vi "Navigation_Main_r1.4 (less sub vis).vi"() -> ()   [LabVIEW 2015]
uses:
  <vilib>/myRIO/Common/Instrument Driver Framework/Utilities/typedefs/Generic FPGA Reference.ctl
  <vilib>/myRIO/Common/Instrument Driver Framework/Utilities/typedefs/myRIO v1.0 Reference.ctl
  <vilib>/myRIO/Common/Instrument Driver Framework/Utilities/typedefs/Hardware Version Enum.ctl
  <vilib>/myRIO/Common/Instrument Driver Framework/Utilities/typedefs/myRIO Generic Hardware Reference.ctl
  <vilib>/userdefined/High Color/nirio_resource_hc.ctl
  <vilib>/myRIO/Instrument Drivers/Onboard IO/PWM/typedefs/PWM Configuration.ctl
  <vilib>/myRIO/Instrument Drivers/Onboard IO/PWM/PWM.lvlib
  <vilib>/myRIO/Common/Instrument Driver Framework/myRIO v1.0/PWM/typedefs/PWM Channels Enum.ctl
  <vilib>/myRIO/Instrument Drivers/Onboard IO/PWM/typedefs/PWM Reference.ctl
  <vilib>/myRIO/Instrument Drivers/Onboard IO/PWM/vis/myRIO PWM Open.xnode
  <vilib>/myRIO/Common/Instrument Driver Framework/myRIO v1.0/PWM/vis/myRIO v1.1 Open PWM.vi
  <vilib>/rvi/interface/nirviOpenFPGA/nirviOpenFPGA.xnode
  <vilib>/myRIO/Instrument Drivers/Utilities/Utilities.lvlib
  <vilib>/rvi/interface/nirviReadWriteControl/nirviReadWriteControl.xnode
  NiFpgaLv.dll
  <vilib>/Utility/error.llb/Error Cluster From Error Code.vi
  <vilib>/rvi/interface/Simulation/niFpgaSimulationCallBeginRW.vi
  <vilib>/rvi/errors/niLvFpgaAdjustHostInterfaceError.vi
  Navi/E/FPGA Bitfiles/NavigationProjec_FPGATarget2_FPGAMainNavigati_PWPHW8gwDxI.lvbitx
  <vilib>/FPGAPlugInAG/myRIO-1900/niLvFpga_Open_myRIO-1900.vi
  <vilib>/rvi/interface/common/dynamic/niFpgaDynamicAddResources.vi
  <vilib>/addons/control/pid/NI_PID_pid.lvlib
  <vilib>/addons/control/pid/pid.llb/PID (DBL).vi
panel:
  out "Avg Right Step":dbl
  out "Avg Left Step":dbl
  out "distance step 2":dbl
  in  "Reset X Y 3":dbl=1.0
  out "Avg Left Dist. New":dbl
  out "Avg Right Dist. New":dbl
  in  "distance step":dbl
  out "step y":dbl
  out "step x":dbl
  out "y traveled new":dbl
  out "x traveled new":dbl
  out "Y traveled old":dbl format="%#_13g"
  out "X traveled old":dbl format="%#_13g"
  out "phi step":dbl
  in  "Reset X Y 2":dbl=1.0
  out "y position":dbl
  out "x position":dbl
  out "phi current":dbl
  out "Phi Current":dbl format="%#_13g"
  out "Desired Y Velocity u2":dbl format="%#_13g"
  out "Desired X Velocity u1":dbl format="%#_13g"
  out "Phi desired":dbl
  out "Omega":dbl format="%.2f"
  out "Desired Velocity":dbl
  in  "omega and angular velocity calc input array 2":dbl[](array[numeric])
  out "robot desired velocity x component\n u1 (ft/s)":dbl
  out "x goal":dbl
  out "x start":dbl
  out "robot desired velocity y component\n u2 (ft/s)":dbl
  out "Y Goal":dbl
  out "Y Position":dbl
  out "Tick Count(mSec) 2":u32 caption="Tick Count(mSec)"
  out "Left Setpoint":dbl
  out "Right Setpoint":dbl
  out "Reset X Y":dbl
  out "Scale":dbl=1.0
  out "x traveled":dbl
  out "v right wheel":dbl
  out "v left wheel":dbl
  out "max v":dbl
  in  "loc_x":dbl
  out "x delta":dbl
  out "x position camera":dbl
  out "encoder step sub vi output":dbl[](array[numeric])
  out "Avg R Dist New":dbl
  out "Avg R Step":dbl
  out "Avg L Dist New":dbl
  out "Avg L Step":dbl
  in  "Avg R Dist Old":dbl
  in  "Avg L Dist Old":dbl
  out "encoder sub vi input array":dbl[](array[numeric])
  out "x & y position output array":dbl[](array[numeric])
  out "x & y position input array":dbl[](array[numeric])
  in  "x traveled old":dbl
  in  "y traveled old":dbl
  in  "phi old":dbl
  in  "Phi Current":dbl format="%#_13g"
  out "Wheel  PID SetPoint input Array":dbl[](array[numeric])
  out "Wheel  PID SetPoint output Array":dbl[](array[numeric])
  in  "Goal Position Y":dbl=5.0
  out "track width(ft)":dbl=4.0
  out "RM Distance (ft)":dbl
  out "RR Distance (ft)":dbl
  out "LF Distance (ft)":dbl
  out "LM Distance (ft)":dbl
  out "RF Distance (ft)":dbl
  out "LR Distance (ft)":dbl
  in  "Start Position Y":dbl=5.0
  in  "Goal Position X":dbl=5.0
  in  "Start Position X":dbl=1.0
  in  "All Stop":bool
  in  "Left Side PID Gains":T1={"proportional gain (Kc)"=0.002, "integral time (Ti, min)"=7e-07, "derivative time (Td, min)"=0.0} {"derivative time (Td, min)" format="%.8f"; "integral time (Ti, min)" format="%.8f"; "proportional gain (Kc)" format="%.8f"}
  in  "Left Side Output Range":cluster{"output high":dbl, "output low":dbl}={"output high"=0.13333, "output low"=-0.13333} {"output low" format="%.5f"; "output high" format="%.5f"}
  in  "Right Side PID Gains":T1={"proportional gain (Kc)"=0.002, "integral time (Ti, min)"=7e-07, "derivative time (Td, min)"=0.0} {"derivative time (Td, min)" format="%.8f"; "integral time (Ti, min)" format="%.8f"; "proportional gain (Kc)" format="%.8f"}
  in  "Right Side Output Range":cluster{"output high":dbl, "output low":dbl}={"output high"=0.13333, "output low"=-0.13333} {"output low" format="%.5f"; "output high" format="%.5f"}
  out "Left PWM":dbl
  out "Right PWM":dbl
  out "LF Rot Velocity (rot/s)":dbl
  out "LM Rot Velocity (rot/s)":dbl
  out "LR Rot Velocity (rot/s)":dbl
  out "RR Rot Velocity (rot/s)":dbl
  out "RM Linear Velocity (rot/s)":dbl
  out "RF Linear Velocity (rot/s)":dbl
  in  "Encoder Reset":bool
  out "SYS.SELECTA":u8 format="%08b"
  out "ENC.B_c.CNTR":i32
  out "ENC.B_b.CNTR":i32
  out "ENC.B_a.CNTR":i32
  out "ENC.A_c.CNTR":i32
  out "ENC.A_b.CNTR":i32
  out "ENC.A_a.CNTR":i32
  out "Current Rot Velocity (rot/s)":T2(graph)
  # "Motor Control Parameters"
  # "Press Go when Start and Goal Are Set"
types:
  T1 = cluster{"proportional gain (Kc)":dbl, "integral time (Ti, min)":dbl, "derivative time (Td, min)":dbl}
  T2 = cluster{"Rotational Velocity (RPS)":dbl, "Rotational Velocity (RPS)":dbl, "Rotational Velocity (RPS)":dbl, "Rotational Velocity (RPS)":dbl, "Rotational Velocity (RPS)":dbl, "Rotational Velocity (RPS)":dbl}
  T3 = typedef "nirio_resource_hc.ctl" = tag
  T4 = typedef "Hardware Version Enum.ctl" = enum16{"Unknown", "myRIO-1900", "myRIO-1950", "roboRIO"}
  T5 = typedef "PWM.lvlib/PWM Reference.ctl" = cluster{"myRIO Reference":T6, "PWM Channels Enum":T9, "PWM Configuration":T10}
  T6 = typedef "myRIO Generic Hardware Reference.ctl" = cluster{"myRIO Model":T4, "myRIO Hardware Reference":T7}
  T7 = typedef "myRIO v1.0 Reference.ctl" = cluster{"Generic FPGA Reference":T8, "Allow multiple opens":bool}
  T8 = typedef "Generic FPGA Reference.ctl" = refnum<k20>
  T9 = typedef "PWM Channels Enum.ctl" = enum16{"Not Connected", "C/PWM0", "C/PWM1", "A/PWM0", "A/PWM1", "A/PWM2", "B/PWM0", "B/PWM1", "B/PWM2", "PWM/PWM0", "PWM/PWM1", "PWM/PWM2", "PWM/PWM3", "PWM/PWM4", "PWM/PWM5", "PWM/PWM6", "PWM/PWM7", "PWM/PWM8", "PWM/PWM9"}
  T10 = typedef "PWM.lvlib/PWM Configuration.ctl" = cluster{"Frequency":dbl, "Duty Cycle":dbl}
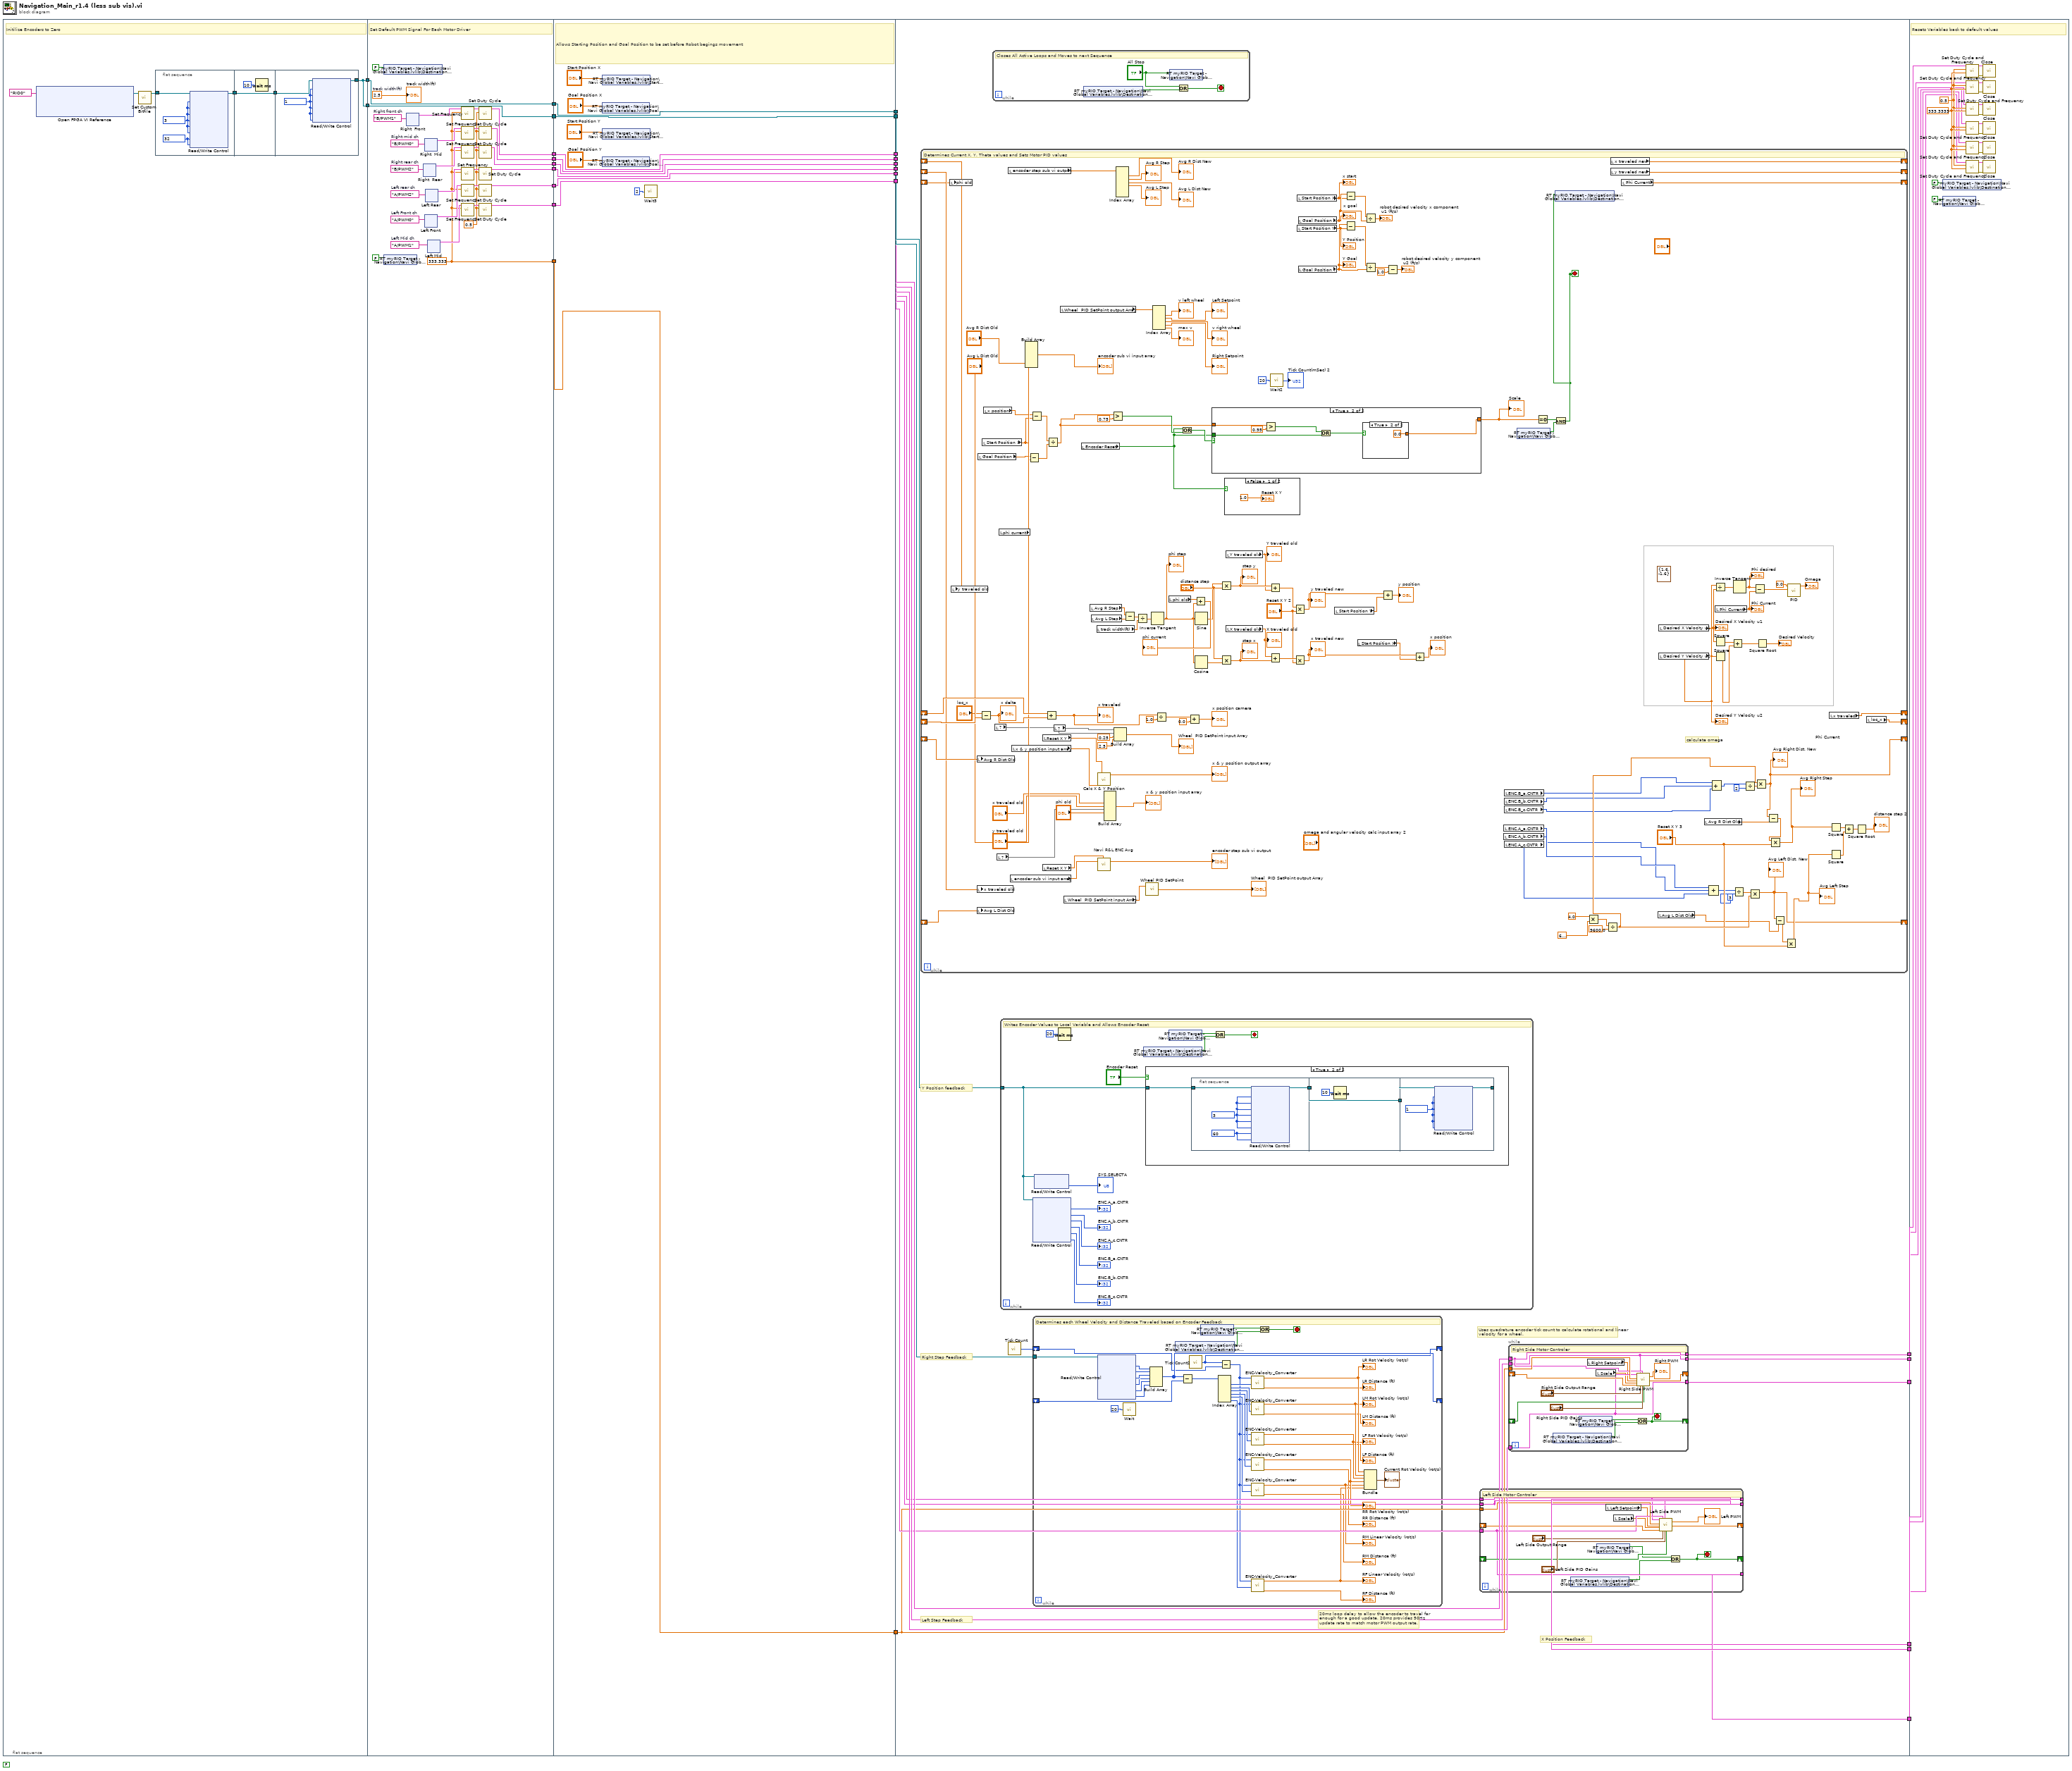
[diagram p0: block diagram]
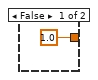
[diagram p2: hidden frame]
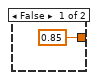
[diagram p3: hidden frame]
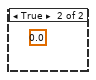
[diagram p4: hidden frame]
diagram:
  (unwired) FALSE ("stop")
  n1 = flat-sequence {
    tunnel: [w29] -> w26
    tunnel: [w29] -> w25
    tunnel: [w60] -> w24
    tunnel: [w55] -> w23
    tunnel: [w51] -> w22
    tunnel: [w50] -> w21
    tunnel: [w49] -> w20
    tunnel: [w48] -> w19
    tunnel: [w47] -> w18
    tunnel: [w46] -> w17
    tunnel: w26 -> [w45]
    tunnel: [w45] -> w16
    tunnel: w25 -> [w46]
    tunnel: w24 -> [w182]
    tunnel: [w182] -> w15
    tunnel: w23 -> [w181]
    tunnel: [w181] -> w14
    tunnel: w22 -> [w180]
    tunnel: [w180] -> w13
    tunnel: w21 -> [w169]
    tunnel: [w169] -> w12
    tunnel: w20 -> [w179]
    tunnel: [w179] -> w11
    tunnel: w19 -> [w178]
    tunnel: [w178] -> w10
    tunnel: w18 -> [w177]
    tunnel: [w177] -> w9
    tunnel: w17 -> [w176]
    tunnel: [w176] -> w8
    tunnel: w16 -> [w175]
    tunnel: [w175] -> w7
    tunnel: w15 -> [w189]
    tunnel: w14 -> [w190]
    tunnel: w13 -> [w195]
    tunnel: w12 -> [w194]
    tunnel: w11 -> [w193]
    tunnel: w10 -> [w192]
    tunnel: w9 -> [w191]
    tunnel: w8 -> [w197]
    tunnel: w7 -> [w196]
    tunnel: [w188] -> w6
    tunnel: [w187] -> w5
    tunnel: [w186] -> w4
    tunnel: [w185] -> w3
    tunnel: [w184] -> w2
    tunnel: [w183] -> w1
    tunnel: w6 -> [w461]
    tunnel: w5 -> [w460]
    tunnel: w4 -> [w459]
    tunnel: w3 -> [w458]
    tunnel: w2 -> [w457]
    tunnel: w1 -> [w456]
    frame #0 {
      # "Initilize Encoders to Zero"
      n2 = xnode "Open FPGA VI Reference"("resource name"=tag "RIO0") -> ("FPGA VI Reference Out"=w28:refnum<k20>)  [unwired: 1 in, 1 out]
      n3 = call <vilib>:"Set Custom Bitfile.vi"("Custom FPGA Reference In"=w28) -> ("Custom FPGA Reference Out"=w30:refnum<k20>)  [unwired: 9 in, 1 out]
      n4 = flat-sequence {
        tunnel: w30 -> [w35]
        tunnel: [w33] -> w32
        tunnel: w32 -> [w37]
        tunnel: [w37] -> w31
        tunnel: w31 -> [w40]
        tunnel: [w39] -> w29
        frame #0 {
          w34 = u8 32 ("SYS.SELECTA")
          w36 = u8 3 ("ENC.B_c.CNFG")
          n5 = xnode "Read/Write Control"("FPGA VI Reference In"=w35, "ENC.A_a.CNFG"=w36, "ENC.A_b.CNFG"=w36, "ENC.A_c.CNFG"=w36, "ENC.B_a.CNFG"=w36, "ENC.B_b.CNFG"=w36, "ENC.B_c.CNFG"=w36, "SYS.SELECTA"=w34, "SYS.SELECTB"=w34) -> ("FPGA VI Reference Out"=w33:refnum<k20>)  [unwired: 1 in, 1 out]
        }
        frame #1 {
          n6 = Wait (ms)(milliseconds to wait=u32 10) -> ()  [unwired: 1 out]
        }
        frame #2 {
          w41 = u8 1 ("ENC.B_c.CNFG")
          n7 = xnode "Read/Write Control"("FPGA VI Reference In"=w40, "ENC.A_a.CNFG"=w41, "ENC.A_b.CNFG"=w41, "ENC.A_c.CNFG"=w41, "ENC.B_a.CNFG"=w41, "ENC.B_b.CNFG"=w41, "ENC.B_c.CNFG"=w41) -> ("FPGA VI Reference Out"=w39:refnum<k20>)  [unwired: 1 in, 1 out]
        }
      }
    }
    frame #1 {
      w42 = 2.5  # track width(ft)
      w52 = 0.5 ("Duty Cycle")
      w60 = 333.333 ("Frequency [Hz]")
      w67 = tag "B/PWM2"  # Right rear ch
      w68 = tag "B/PWM0"  # Right mid ch
      w69 = tag "B/PWM1"  # Right front ch
      w70 = tag "A/PWM2"  # Left rear ch
      w71 = tag "A/PWM0"  # Left Front ch
      w72 = tag "A/PWM1"  # Left Mid ch
      # "Set Default PWM Signal For Each Motor Driver"
      n8 = shared-variable "RT myRIO Target - Navigation\\Navi Global Variables.lvlib\\Destination Reached"(FALSE) -> ()  [unwired: 1 in, 1 out]
      n9 = shared-variable "RT myRIO Target - Navigation\\Navi Global Variables.lvlib\\All Stop"(FALSE) -> ()  [unwired: 1 in, 1 out]
      n10 = xnode "Right  Front"("Channel Name"=w69) -> ("PWM Ref Out"=w63:T5)  [unwired: 2 in, 1 out]
      n11 = xnode "Right  Rear"("Channel Name"=w67) -> ("PWM Ref Out"=w61:T5)  [unwired: 2 in, 1 out]
      n12 = xnode "Right  Mid"("Channel Name"=w68) -> ("PWM Ref Out"=w62:T5)  [unwired: 2 in, 1 out]
      n13 = xnode "Left Front"("Channel Name"=w71) -> ("PWM Ref Out"=w65:T5)  [unwired: 2 in, 1 out]
      n14 = xnode "Left Rear"("Channel Name"=w70) -> ("PWM Ref Out"=w64:T5)  [unwired: 2 in, 1 out]
      n15 = xnode "Left Mid"("Channel Name"=w72) -> ("PWM Ref Out"=w66:T5)  [unwired: 2 in, 1 out]
      n16 = call <vilib>:"Set Frequency.vi"("Frequency [Hz]"=w60, "PWM Ref In"=w63) -> ("PWM Ref Out"=w56:T5)  [unwired: 7 in, 1 out]
      n17 = call <vilib>:"Set Frequency.vi"("Frequency [Hz]"=w60, "PWM Ref In"=w62) -> ("PWM Ref Out"=w57:T5)  [unwired: 7 in, 1 out]
      n18 = call <vilib>:"Set Frequency.vi"("Frequency [Hz]"=w60, "PWM Ref In"=w61) -> ("PWM Ref Out"=w58:T5)  [unwired: 7 in, 1 out]
      n19 = call <vilib>:"Set Frequency.vi"("Frequency [Hz]"=w60, "PWM Ref In"=w64) -> ("PWM Ref Out"=w54:T5)  [unwired: 7 in, 1 out]
      n20 = call <vilib>:"Set Frequency.vi"("Frequency [Hz]"=w60, "PWM Ref In"=w65) -> ("PWM Ref Out"=w53:T5)  [unwired: 7 in, 1 out]
      n21 = call <vilib>:"Set Frequency.vi"("Frequency [Hz]"=w60, "PWM Ref In"=w66) -> ("PWM Ref Out"=w59:T5)  [unwired: 7 in, 1 out]
      n22 = call <vilib>:"Set Duty Cycle.vi"("Duty Cycle"=w52, "PWM Ref In"=w56) -> ("PWM Ref Out"=w51:T5)  [unwired: 7 in, 1 out]
      n23 = call <vilib>:"Set Duty Cycle.vi"("Duty Cycle"=w52, "PWM Ref In"=w57) -> ("PWM Ref Out"=w50:T5)  [unwired: 7 in, 1 out]
      n24 = call <vilib>:"Set Duty Cycle.vi"("Duty Cycle"=w52, "PWM Ref In"=w58) -> ("PWM Ref Out"=w49:T5)  [unwired: 7 in, 1 out]
      n25 = call <vilib>:"Set Duty Cycle.vi"("Duty Cycle"=w52, "PWM Ref In"=w54) -> ("PWM Ref Out"=w55:T5)  [unwired: 7 in, 1 out]
      n26 = call <vilib>:"Set Duty Cycle.vi"("Duty Cycle"=w52, "PWM Ref In"=w53) -> ("PWM Ref Out"=w48:T5)  [unwired: 7 in, 1 out]
      n27 = call <vilib>:"Set Duty Cycle.vi"("Duty Cycle"=w52, "PWM Ref In"=w59) -> ("PWM Ref Out"=w47:T5)  [unwired: 7 in, 1 out]
      "track width(ft)" <- w42
    }
    frame #2 {
      # "Allows Starting Position and Goal Position to be set before Robot begings movement"
      n28 = shared-variable "RT myRIO Target - Navigation\\Navi Global Variables.lvlib\\Start Position X"("Start Position X") -> ()  [unwired: 1 in, 1 out]
      n29 = shared-variable "RT myRIO Target - Navigation\\Navi Global Variables.lvlib\\Goal Position X"("Goal Position X") -> ()  [unwired: 1 in, 1 out]
      n30 = shared-variable "RT myRIO Target - Navigation\\Navi Global Variables.lvlib\\Start Position Y"("Start Position Y") -> ()  [unwired: 1 in, 1 out]
      n31 = shared-variable "RT myRIO Target - Navigation\\Navi Global Variables.lvlib\\Goal Position Y"("Goal Position Y") -> ()  [unwired: 1 in, 1 out]
      n32 = call "Wait3"("Count(mSec)"=u32 2) -> ()  [unwired: 1 out]
    }
    frame #3 {
      # "Left Step Feedback"
      # "Y Position feedback"
      # "Right Step Feedback"
      # "X Position Feedback"
      # "Uses quadrature encoder tick count to calculate rotational and linear velocity for a wheel."
      # "20ms loop delay to allow the encoder to travel far enough for a good update. 20ms provides 50Hz update rate to match motor PWM output rate."
      n33 = while {
        shift-right: [w339] -> _
        shift-left: _ -> [w340]
        shift-right: [w336] -> _
        shift-left: _ -> [w337]
        shift-right: [w202] -> _
        shift-left: _ -> [w321]
        shift-right: [w200] -> _
        shift-left: _ -> [w322]
        shift-right: [w310] -> _
        shift-left: _ -> [w304]
        shift-right: [w311] -> _
        shift-left: _ -> [w305]
        shift-right: [w312] -> _
        shift-left: _ -> [w303]
        stop <- w284 stop-if-true
        (unwired) cluster{"output high":dbl, "output low":dbl} {"output high"=1.6, "output low"=-1.6} ("output range")
        # "calculate omega"
        # "Determines Current X, Y, Theta values and Sets Motor PID values"
        n34 = local write "phi old"(w303) -> ()
        n35 = local write "y traveled old"(w304) -> ()
        n36 = local write "Avg R Dist Old"(w322) -> ()
        n37 = local write "x traveled old"(w305) -> ()
        n38 = local write "Avg L Dist Old"(w321) -> ()
        n39 = local read "Goal Position X"() -> (w235:dbl)
        n40 = Subtract(x="loc_x", y=w340) -> (x-y=w338:dbl)
        "x delta" <- w338
        n41 = local read "Start Position X"() -> (w236:dbl)
        n42 = local read "x position"() -> (w237:dbl)
        n43 = local read item#-1() -> (w300)
        n44 = local read item#-1() -> (w307)
        n45 = local read "phi current"() -> ()  [unwired: 1 out]
        n46 = local read "encoder step sub vi output"() -> (w325:dbl[])
        n47 = local read "encoder sub vi input array"() -> (w330:dbl[])
        n48 = local read "x & y position input array"() -> (w302:dbl[])
        n49 = Build Array("Avg R Dist Old", "Avg L Dist Old") -> (→"encoder sub vi input array":dbl[], w211:dbl, w210:dbl, w315:dbl, w316:dbl, w317:dbl, w209:dbl)
        n50 = Subtract(x=w235, y=w236) -> (x-y=w233:dbl)
        n51 = Subtract(x=w237, y=w236) -> (x-y=w234:dbl)
        n52 = local read "Reset X Y"() -> (w301:dbl)
        n53 = local read "Reset X Y"() -> (w331:dbl)
        n54 = Add(x=w337, y=w338) -> (x+y=w335:dbl)
        "x traveled" <- w335
        n55 = Divide(x=w234, y=w233) -> (x/y=w232:dbl)
        n56 = local read item#-1() -> (w299)
        n57 = local read "Wheel  PID SetPoint output Array"() -> (w293:dbl[])
        n58 = local read "Wheel  PID SetPoint input Array"() -> (w295:dbl[])
        n59 = local read "Encoder Reset"() -> (w341:bool)
        n60 = local read "Avg R Step"() -> (w245:dbl)
        n61 = local read "Avg L Step"() -> (w244:dbl)
        n62 = local read "track width(ft)"() -> (w243:dbl)
        n63 = call "Calc X & Y Position.vi"("x & y position input array"=w302, "Reset X Y"=w301) -> ("y & x traveled output array"=→"x & y position output array":dbl[])  [unwired: 16 in, 1 out]
        n64 = call "Navi R&L ENC Avg.vi"("encoder step sub vi input"=w330, "Reset X Y"=w331) -> ("encoder step sub vi output"=→"encoder step sub vi output":dbl[])  [unwired: 17 in]
        n65 = Build Array("x traveled old", "y traveled old", w307, "phi old") -> (→"x & y position input array":dbl[])  [unwired: 5 in]
        n66 = Greater?(x=w232, y=0.75) -> (0:w342:bool)
        n67 = Build Array(w299, w300, 0.25 ("element"), 2.5 ("element")) -> (→"Wheel  PID SetPoint input Array":dbl[])
        n68 = Index Array(array=w325) -> (element #1=→"Avg R Dist New":dbl, element #2=→"Avg R Step":dbl, element #3=→"Avg L Dist New":dbl, element #4=→"Avg L Step":dbl, element #5=w328:dbl)  [unwired: 7 in, 2 out]
        n69 = Subtract(x=w245, y=w244) -> (x-y=w250:dbl)
        n70 = Divide(x=w250, y=w243) -> (x/y=w251:dbl)
        n71 = call "Wheel PID SetPoint.vi"("Wheel  PID SetPoint Input Array"=w295) -> ("Wheel  PID SetPoint output Array"=→"Wheel  PID SetPoint output Array":dbl[])  [unwired: 1 in]
        n72 = Inverse Tangent(1:w251) -> (0:w260:dbl)
        "phi step" <- w260
        n73 = Index Array(array=w293) -> (element #1=→"v left wheel":dbl, element #2=→"Left Setpoint":dbl, element #3=→"v right wheel":dbl, element #4=→"Right Setpoint":dbl, element #5=→"max v":dbl)  [unwired: 5 in]
        n74 = Divide(x=w335, y=1.0) -> (x/y=w333:dbl)
        n75 = local read "phi old"() -> (w242:dbl)
        n76 = Or(x=w341, y=w342) -> (x .or. y?=w343:bool)
        n77 = Add(x=w333, y=0.0) -> (x+y=→"x position camera":dbl)
        n78 = Add(x=w242, y=w260) -> (x+y=→"phi current":dbl)
        n79 = Sine(x=w260) -> (sin(x)=w249:dbl)
        n80 = Cosine(x=w260) -> (cos(x)=w248:dbl)
        n81 = case shown="True" w343 {
          tunnel: w232 -> [_ w355]
          tunnel: [1.0 w352] -> w344
          tunnel: w341 -> [_ w350]
          frame False {
          }
          frame True {
            n82 = Greater?(x=w355, y=0.95) -> (0:w353:bool)
            n83 = Or(x=w353, y=w350) -> (x .or. y?=w351:bool)
            n84 = case shown="True" w351 {
              tunnel: [0.85 0.0] -> w352
              frame False {
              }
              frame True {
              }
            }
          }
        }
        "Scale" <- w344
        n85 = Multiply(x=w249, y="distance step") -> (x*y=w247:dbl)
        "step y" <- w247
        n86 = Multiply(x="distance step", y=w248) -> (x*y=w246:dbl)
        "step x" <- w246
        n87 = case shown="False" w341 {
          frame False {
            "Reset X Y" <- 1.0
          }
          frame True {
            w359 = 0.0
          }
        }
        n88 = local read "Y traveled old"() -> (w241:dbl)
        "Y traveled old" <- w241
        n89 = local read "X traveled old"() -> (w240:dbl)
        "X traveled old" <- w240
        n90 = Add(x=w247, y=w241) -> (x+y=w254:dbl)
        n91 = Add(x=w240, y=w246) -> (x+y=w253:dbl)
        n92 = call "Wait2"("Count(mSec)"=u32 20) -> ("Tick Count(mSec)"=→"Tick Count(mSec) 2":u32)
        n93 = Multiply(x=w254, y="Reset X Y 2") -> (x*y=w255:dbl)
        "y traveled new" <- w255
        n94 = Multiply(x=w253, y="Reset X Y 2") -> (x*y=w257:dbl)
        "x traveled new" <- w257
        n95 = local read "Start Position X"() -> (w274:dbl)
        "x start" <- w274
        n96 = local read "Start Position Y"() -> (w279:dbl)
        "Y Position" <- w279
        n97 = local read "Goal Position X"() -> (w275:dbl)
        "x goal" <- w275
        n98 = local read "Goal Position Y"() -> (w278:dbl)
        "Y Goal" <- w278
        n99 = local read "Start Position Y"() -> (w239:dbl)
        n100 = Subtract(x=w275, y=w274) -> (x-y=w277:dbl)
        n101 = Subtract(x=w278, y=w279) -> (x-y=w280:dbl)
        n102 = local read "Start Position X"() -> (w238:dbl)
        n103 = Divide(x=w277, y=w275) -> (x/y=→"robot desired velocity x component\n u1 (ft/s)":dbl)
        n104 = Divide(x=w280, y=w278) -> (x/y=w281:dbl)
        n105 = Add(x=w255, y=w239) -> (x+y=→"y position":dbl)
        n106 = Subtract(x=w281, y=1.0) -> (x-y=→"robot desired velocity y component\n u2 (ft/s)":dbl)
        n107 = Add(x=w257, y=w238) -> (x+y=→"x position":dbl)
        n108 = local read "ENC.A_a.CNTR"() -> (w205:i32)
        n109 = local read "ENC.A_b.CNTR"() -> (w204:i32)
        n110 = local read "ENC.B_a.CNTR"() -> (w208:i32)
        n111 = local read "ENC.B_b.CNTR"() -> (w207:i32)
        n112 = local read "ENC.B_c.CNTR"() -> (w206:i32)
        n113 = local read "ENC.A_c.CNTR"() -> (w203:i32)
        n114 = shared-variable "RT myRIO Target - Navigation\\Navi Global Variables.lvlib\\All Stop"() -> (w346:bool)  [unwired: 1 in, 1 out]
        n115 = Equal To 0?(x=w344) -> (x = 0?=w285:bool)
        n116 = And(x=w285, y=w346) -> (x .and. y?=w284:bool)
        n117 = shared-variable "RT myRIO Target - Navigation\\Navi Global Variables.lvlib\\Destination Reached"(w284) -> ()  [unwired: 1 in, 1 out]
        n118 = Multiply(x=4.0, y=6.283185307179586) -> (x*y=w230:dbl)
        n119 = Divide(x=w230, y=9600.0) -> (x/y=w231:dbl)
        n120 = local read "x traveled new"() -> (w310:dbl)
        n121 = local read "y traveled new"() -> (w311:dbl)
        n122 = local read "Phi Current"() -> (w312:dbl)
        n123 = local read "Avg L Dist Old"() -> (w201:dbl)
        n124 = local read "Desired X Velocity u1"() -> (w263:dbl)
        "Desired X Velocity u1" <- w263
        n125 = local read "Desired Y Velocity u2"() -> (w264:dbl)
        "Desired Y Velocity u2" <- w264
        n126 = local read "Avg R Dist Old"() -> (w199:dbl)
        n127 = Compound Arithmetic op=ADD(w205, w204, w203) -> (w214:i32)
        n128 = Compound Arithmetic op=ADD(w208, w207, w206) -> (w212:i32)
        n129 = Divide(x=w264, y=w263) -> (x/y=w265:dbl)
        n130 = Square(x=w263) -> (x^2=w266:dbl)
        n131 = Square(x=w264) -> (x^2=w267:dbl)
        n132 = local read "Phi Current"() -> (w262:dbl)
        "Phi Current" <- w262
        n133 = Add(x=w266, y=w267) -> (x+y=w268:dbl)
        n134 = Divide(x=w214, y=3) -> (x/y=w226:dbl)
        n135 = Inverse Tangent(1:w265) -> (0:w270:dbl)
        "Phi desired" <- w270
        n136 = Divide(x=w212, y=2) -> (x/y=w223:dbl)
        n137 = Multiply(x=w226, y=w231) -> (x*y=w202:dbl)
        "Avg Left Dist. New" <- w202
        n138 = Subtract(x=w270, y=w262) -> (x-y=w272:dbl)
        n139 = Multiply(x=w231, y=w223) -> (x*y=w200:dbl)
        "Avg Right Dist. New" <- w200
        n140 = Square Root(x=w268) -> (sqrt(x)=→"Desired Velocity":dbl)
        n141 = Subtract(x=w200, y=w199) -> (x-y=w221:dbl)
        n142 = Multiply(x=w221, y="Reset X Y 3") -> (x*y=w224:dbl)
        "Avg Right Step" <- w224
        n143 = Subtract(x=w202, y=w201) -> (x-y=w222:dbl)
        n144 = Multiply(x=w222, y="Reset X Y 3") -> (x*y=w225:dbl)
        "Avg Left Step" <- w225
        n145 = call-poly <vilib>:"PID.vi"("process variable"=w272, "setpoint"=0.0) -> ("output"=→"Omega":dbl)  [unwired: 8 in, 1 out]
        n146 = local read "x traveled"() -> (w336:dbl)
        n147 = Square(x=w224) -> (x^2=w218:dbl)
        n148 = Square(x=w225) -> (x^2=w219:dbl)
        n149 = Add(x=w218, y=w219) -> (x+y=w217:dbl)
        n150 = Square Root(x=w217) -> (sqrt(x)=→"distance step 2":dbl)
        n151 = local read "loc_x"() -> (w339:dbl)
      }
      n152 = while {
        stop <- w362 stop-if-true
        # "Closes All Active Loops and Moves to next Sequence"
        n153 = shared-variable "RT myRIO Target - Navigation\\Navi Global Variables.lvlib\\Destination Reached"() -> (w360:bool)  [unwired: 1 in, 1 out]
        n154 = shared-variable "RT myRIO Target - Navigation\\Navi Global Variables.lvlib\\All Stop"("All Stop") -> ()  [unwired: 1 in, 1 out]
        n155 = Or(x="All Stop", y=w360) -> (x .or. y?=w362:bool)
      }
      n156 = while {
        tunnel: w197 -> [w396]
        stop <- w393 stop-if-true
        # "Writes Encoder Values to Local Variable and Allows Encoder Reset"
        n157 = xnode "Read/Write Control"("FPGA VI Reference In"=w396) -> ("ENC.A_a.CNTR"=→"ENC.A_a.CNTR":u32, "ENC.A_b.CNTR"=→"ENC.A_b.CNTR":u32, "ENC.A_c.CNTR"=→"ENC.A_c.CNTR":u32, "ENC.B_a.CNTR"=→"ENC.B_a.CNTR":u32, "ENC.B_b.CNTR"=→"ENC.B_b.CNTR":u32, "ENC.B_c.CNTR"=→"ENC.B_c.CNTR":u32)  [unwired: 1 in, 2 out]
        n158 = xnode "Read/Write Control"("FPGA VI Reference In"=w396) -> ("SYS.SELECTA"=→"SYS.SELECTA":u8)  [unwired: 1 in, 2 out]
        n159 = Wait (ms)(milliseconds to wait=u32 20) -> ()  [unwired: 1 out]
        n160 = shared-variable "RT myRIO Target - Navigation\\Navi Global Variables.lvlib\\Destination Reached"() -> (w395:bool)  [unwired: 1 in, 1 out]
        n161 = case shown="True" "Encoder Reset" {
          tunnel: w396 -> [_ w406]
          frame False {
          }
          frame True {
            n162 = flat-sequence {
              tunnel: w406 -> [w411]
              tunnel: [w409] -> w408
              tunnel: w408 -> [w413]
              tunnel: [w413] -> w407
              tunnel: w407 -> [w416]
              tunnel: [w415] -> _
              frame #0 {
                w410 = u8 60 ("SYS.SELECTA")
                w412 = u8 3 ("ENC.B_c.CNFG")
                n163 = xnode "Read/Write Control"("FPGA VI Reference In"=w411, "ENC.A_a.CNFG"=w412, "ENC.A_b.CNFG"=w412, "ENC.A_c.CNFG"=w412, "ENC.B_a.CNFG"=w412, "ENC.B_b.CNFG"=w412, "ENC.B_c.CNFG"=w412, "SYS.SELECTA"=w410, "SYS.SELECTB"=w410) -> ("FPGA VI Reference Out"=w409:refnum<k20>)  [unwired: 1 in, 1 out]
              }
              frame #1 {
                n164 = Wait (ms)(milliseconds to wait=u32 10) -> ()  [unwired: 1 out]
              }
              frame #2 {
                w417 = u8 1 ("ENC.B_c.CNFG")
                n165 = xnode "Read/Write Control"("FPGA VI Reference In"=w416, "ENC.A_a.CNFG"=w417, "ENC.A_b.CNFG"=w417, "ENC.A_c.CNFG"=w417, "ENC.B_a.CNFG"=w417, "ENC.B_b.CNFG"=w417, "ENC.B_c.CNFG"=w417) -> ("FPGA VI Reference Out"=w415:refnum<k20>)  [unwired: 1 in, 1 out]
              }
            }
          }
        }
        n166 = shared-variable "RT myRIO Target - Navigation\\Navi Global Variables.lvlib\\All Stop"() -> (w394:bool)  [unwired: 1 in, 1 out]
        n167 = Or(x=w394, y=w395) -> (x .or. y?=w393:bool)
      }
      n168 = call "Tick Count"() -> ("Tick Count(uSec)"=w198:u32)
      n169 = while {
        shift-right: [w445] -> _
        shift-left: _ -> [w444]
        shift-right: [w442] -> _
        shift-left: w198 -> [w441]
        tunnel: w196 -> [w452]
        stop <- w437 stop-if-true
        # "Determines each Wheel Velocity and Distance Traveled based on Encoder Feedback"
        n170 = xnode "Read/Write Control"("FPGA VI Reference In"=w452) -> ("ENC.A_a.CNTR"=w451:u32, "ENC.A_b.CNTR"=w450:u32, "ENC.A_c.CNTR"=w449:u32, "ENC.B_a.CNTR"=w448:u32, "ENC.B_b.CNTR"=w447:u32, "ENC.B_c.CNTR"=w446:u32)  [unwired: 1 in, 2 out]
        n171 = call "Wait"("Count(mSec)"=u32 20) -> ()  [unwired: 1 out]
        n172 = Build Array(w451, w450, w449, w448, w447, w446) -> (w445:u32[])
        n173 = shared-variable "RT myRIO Target - Navigation\\Navi Global Variables.lvlib\\Destination Reached"() -> (w439:bool)  [unwired: 1 in, 1 out]
        n174 = Subtract(x=w445, y=w444) -> (x-y=w443:u32[])
        n175 = call "Tick Count2"() -> ("Tick Count(uSec)"=w442:u32)
        n176 = shared-variable "RT myRIO Target - Navigation\\Navi Global Variables.lvlib\\All Stop"() -> (w438:bool)  [unwired: 1 in, 1 out]
        n177 = Index Array(array=w443) -> (element #1=w436:u32, element #2=w433:u32, element #3=w431:u32, element #4=w429:u32, element #5=w427:u32, element #6=w424:u32)  [unwired: 6 in]
        n178 = Subtract(x=w442, y=w441) -> (x-y=w425:u32)
        n179 = call "ENC-Velocity_Converter.vi"("delta  Encoder Count"=w436, "dt (uSec)"=w425) -> ("Distance (ft)"=→"LR Distance (ft)":dbl, "Rotational Velocity (RPS)"=w435:dbl)  [unwired: 7 in, 1 out]
        "LR Rot Velocity (rot/s)" <- w435
        n180 = call "ENC-Velocity_Converter.vi"("delta  Encoder Count"=w433, "dt (uSec)"=w425) -> ("Distance (ft)"=→"LM Distance (ft)":dbl, "Rotational Velocity (RPS)"=w434:dbl)  [unwired: 7 in, 1 out]
        "LM Rot Velocity (rot/s)" <- w434
        n181 = call "ENC-Velocity_Converter.vi"("delta  Encoder Count"=w431, "dt (uSec)"=w425) -> ("Distance (ft)"=→"LF Distance (ft)":dbl, "Rotational Velocity (RPS)"=w432:dbl)  [unwired: 7 in, 1 out]
        "LF Rot Velocity (rot/s)" <- w432
        n182 = call "ENC-Velocity_Converter.vi"("delta  Encoder Count"=w429, "dt (uSec)"=w425) -> ("Distance (ft)"=→"RR Distance (ft)":dbl, "Rotational Velocity (RPS)"=w430:dbl)  [unwired: 7 in, 1 out]
        "RR Rot Velocity (rot/s)" <- w430
        n183 = call "ENC-Velocity_Converter.vi"("delta  Encoder Count"=w427, "dt (uSec)"=w425) -> ("Distance (ft)"=→"RM Distance (ft)":dbl, "Rotational Velocity (RPS)"=w428:dbl)  [unwired: 7 in, 1 out]
        "RM Linear Velocity (rot/s)" <- w428
        n184 = call "ENC-Velocity_Converter.vi"("delta  Encoder Count"=w424, "dt (uSec)"=w425) -> ("Distance (ft)"=→"RF Distance (ft)":dbl, "Rotational Velocity (RPS)"=w426:dbl)  [unwired: 7 in, 1 out]
        "RF Linear Velocity (rot/s)" <- w426
        n185 = Or(x=w438, y=w439) -> (x .or. y?=w437:bool)
        n186 = Bundle("Rotational Velocity (RPS)"=w435, "Rotational Velocity (RPS)"=w434, "Rotational Velocity (RPS)"=w432, "Rotational Velocity (RPS)"=w430, "Rotational Velocity (RPS)"=w428, "Rotational Velocity (RPS)"=w426) -> (→"Current Rot Velocity (rot/s)":T2)  [unwired: 1 in]
      }
      n187 = while {
        tunnel: w192 -> [w370]
        tunnel: w191 -> [w369]
        tunnel: w190 -> [w368]
        tunnel: w189 -> [w377]
        shift-right: [w373] -> _
        shift-left: _ -> [w372]
        shift-right: [w365] -> _
        shift-left: _ -> [w371]
        tunnel: [w370] -> w185
        tunnel: [w369] -> w184
        tunnel: [w368] -> w183
        stop <- w365 stop-if-true
        # "Left Side Motor Controler"
        n188 = shared-variable "RT myRIO Target - Navigation\\Navi Global Variables.lvlib\\Destination Reached"() -> (w367:bool)  [unwired: 1 in, 1 out]
        n189 = shared-variable "RT myRIO Target - Navigation\\Navi Global Variables.lvlib\\All Stop"() -> (w366:bool)  [unwired: 1 in, 1 out]
        n190 = local read "Left Setpoint"() -> (w364:dbl)
        n191 = local read "Scale"() -> (w363:dbl)
        n192 = call "Left Side PWM.vi"("Left rear"=w368, "Frequency"=w377, "Left Side Setpoint"=w364, "Left Side Scale"=w363, "Left PID Feedback"=w372, "Left Mid"=w369, "Left Side Output Range"="Left Side Output Range", "Left Front"=w370, "Left Side PID Gains"="Left Side PID Gains", "Reset Left E.T."=w371) -> ("Left PWM"=→"Left PWM":dbl, "Left PID Output"=w373:dbl)  [unwired: 8 in]
        n193 = Or(x=w366, y=w367) -> (x .or. y?=w365:bool)
      }
      n194 = while {
        tunnel: w195 -> [w385]
        tunnel: w194 -> [w384]
        tunnel: w193 -> [w383]
        tunnel: w189 -> [w392]
        shift-right: [w388] -> _
        shift-left: _ -> [w387]
        shift-right: [w380] -> _
        shift-left: _ -> [w386]
        tunnel: [w385] -> w188
        tunnel: [w384] -> w187
        tunnel: [w383] -> w186
        stop <- w380 stop-if-true
        # "Right Side Motor Controler"
        n195 = shared-variable "RT myRIO Target - Navigation\\Navi Global Variables.lvlib\\Destination Reached"() -> (w382:bool)  [unwired: 1 in, 1 out]
        n196 = shared-variable "RT myRIO Target - Navigation\\Navi Global Variables.lvlib\\All Stop"() -> (w381:bool)  [unwired: 1 in, 1 out]
        n197 = local read "Right Setpoint"() -> (w379:dbl)
        n198 = local read "Scale"() -> (w378:dbl)
        n199 = Or(x=w381, y=w382) -> (x .or. y?=w380:bool)
        n200 = call "Right Side PWM.vi"("Right rear"=w383, "Frequency"=w392, "Right Side Setpoint"=w379, "Right Side Scale"=w378, "Right PID Feedback"=w387, "Right Mid"=w384, "Right Side Output Range"="Right Side Output Range", "Right Front"=w385, "Right Side PID Gains"="Right Side PID Gains", "Reset Right E.T."=w386) -> ("Right PWM"=→"Right PWM":dbl, "Right PID Output"=w388:dbl)  [unwired: 8 in]
      }
    }
    frame #4 {
      w462 = 0.5
      w463 = 333.3333
      # "Resets Variables back to default values"
      n201 = shared-variable "RT myRIO Target - Navigation\\Navi Global Variables.lvlib\\Destination Reached"(FALSE) -> ()  [unwired: 1 in, 1 out]
      n202 = shared-variable "RT myRIO Target - Navigation\\Navi Global Variables.lvlib\\All Stop"(FALSE) -> ()  [unwired: 1 in, 1 out]
      n203 = call <vilib>:"Set Duty Cycle and Frequency.vi"("Frequency [Hz]"=w463, "Duty Cycle"=w462, "PWM Ref In"=w461) -> ("error out"=w468:errorcluster, "PWM Ref Out"=w475:T5)  [unwired: 6 in]
      n204 = call <vilib>:"Set Duty Cycle and Frequency.vi"("Frequency [Hz]"=w463, "Duty Cycle"=w462, "PWM Ref In"=w460) -> ("error out"=w473:errorcluster, "PWM Ref Out"=w474:T5)  [unwired: 6 in]
      n205 = call <vilib>:"Set Duty Cycle and Frequency.vi"("Frequency [Hz]"=w463, "Duty Cycle"=w462, "PWM Ref In"=w459) -> ("error out"=w467:errorcluster, "PWM Ref Out"=w472:T5)  [unwired: 6 in]
      n206 = call <vilib>:"Set Duty Cycle and Frequency.vi"("Frequency [Hz]"=w463, "Duty Cycle"=w462, "PWM Ref In"=w456) -> ("error out"=w464:errorcluster, "PWM Ref Out"=w469:T5)  [unwired: 6 in]
      n207 = call <vilib>:"Set Duty Cycle and Frequency.vi"("Frequency [Hz]"=w463, "Duty Cycle"=w462, "PWM Ref In"=w458) -> ("error out"=w466:errorcluster, "PWM Ref Out"=w471:T5)  [unwired: 6 in]
      n208 = call <vilib>:"Set Duty Cycle and Frequency.vi"("Frequency [Hz]"=w463, "Duty Cycle"=w462, "PWM Ref In"=w457) -> ("error out"=w465:errorcluster, "PWM Ref Out"=w470:T5)  [unwired: 6 in]
      n209 = call <vilib>:"Close.vi"("error in (no error)"=w468, "PWM Ref In"=w475) -> ()  [unwired: 9 in, 1 out]
      n210 = call <vilib>:"Close.vi"("error in (no error)"=w473, "PWM Ref In"=w474) -> ()  [unwired: 9 in, 1 out]
      n211 = call <vilib>:"Close.vi"("error in (no error)"=w467, "PWM Ref In"=w472) -> ()  [unwired: 9 in, 1 out]
      n212 = call <vilib>:"Close.vi"("error in (no error)"=w464, "PWM Ref In"=w469) -> ()  [unwired: 9 in, 1 out]
      n213 = call <vilib>:"Close.vi"("error in (no error)"=w466, "PWM Ref In"=w471) -> ()  [unwired: 9 in, 1 out]
      n214 = call <vilib>:"Close.vi"("error in (no error)"=w465, "PWM Ref In"=w470) -> ()  [unwired: 9 in, 1 out]
    }
  }
